vi "MBtcp-WriteCoil.vi"() -> ()   [LabVIEW 2022 SP3]
uses:
  <vilib>/Plasmionique/MB Master/MB_Master_TCP/MB_Master_TCP.lvclass
  Applications/National Instruments/LabVIEW 2022 64-bit/vi.lib/Plasmionique/MB Master/MB_Master/MB_Master.lvclass
  <vilib>/Plasmionique/MB Master/MB Master.lvlib
panel:
  in  "Slave ID":u8=255 format="%.0x"
  in  "value":bool
  out "error out":errorcluster
  in  "IP Address":string
  in  "RegisterAddr":u16
  in  "error in (no error)":errorcluster
  in  "Port":u16=502
  in  "Timeout (900)":i32=900
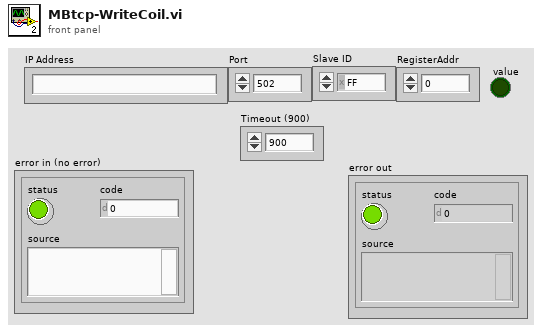
[diagram p1: front panel]
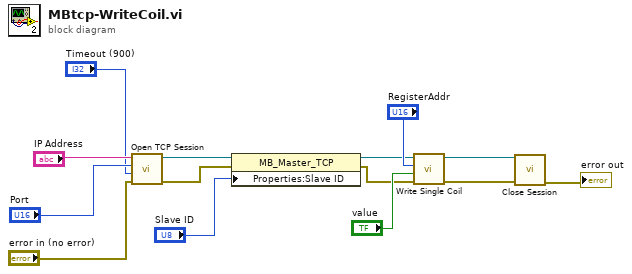
[diagram p0: block diagram]
diagram:
  n1 = call <vilib>:"Open TCP Session.vi"("error in (no error)"="error in (no error)", "Timeout (10000)"="Timeout (900)", "Port (502)"="Port", "IP Address"="IP Address") -> ("error out"=w3:errorcluster, "MB_TCP session"=w14:refnum<class "MB_Master_TCP.lvclass">)  [unwired: 6 in]
  n2 = property class="MB_Master_TCP"(reference=w14, error in=w3, "Properties:Slave ID"="Slave ID") -> (reference out=w4:refnum<class "MB_Master_TCP.lvclass">, error out=w2:errorcluster)
  n3 = call <vilib>:"Write Single Coil.vi"("error in (no error)"=w2, "value"="value", "address"="RegisterAddr", "MB session in"=w4) -> ("error out"=w12:errorcluster, "MB session out"=w13:refnum<class "MB_Master_TCP.lvclass">)  [unwired: 6 in]
  n4 = call-dynamic "Close Session.vi"("error in (no error)"=w12, "MB TCP session"=w13) -> ("error out"=→"error out":errorcluster)  [unwired: 9 in]
